vi "example.vi"() -> ()   [LabVIEW 2025, in "Dynamic-System.lvclass"]
uses:
  Dynamic-System.lvclass
  controller selection.ctl
panel:
  out "XY Graph":cluster{"Time":dbl[], "Reference":dbl[]}[](graph)
  in  "stop":bool
  out "error out":errorcluster
  out "Dynamic-System out":refnum<class "Dynamic-System.lvclass">
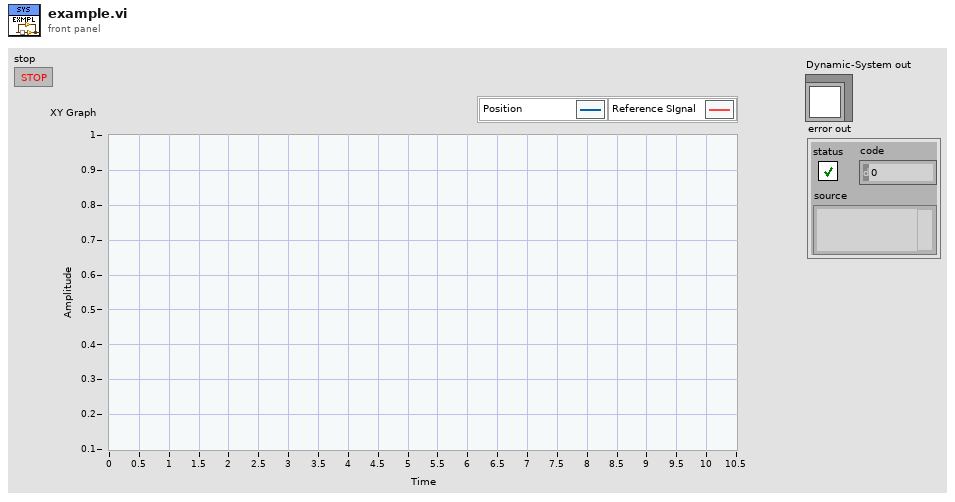
[diagram p1: front panel]
types:
  T1 = typedef "controller selection.ctl" = enum16{"No Control", "PID", "On Off"}
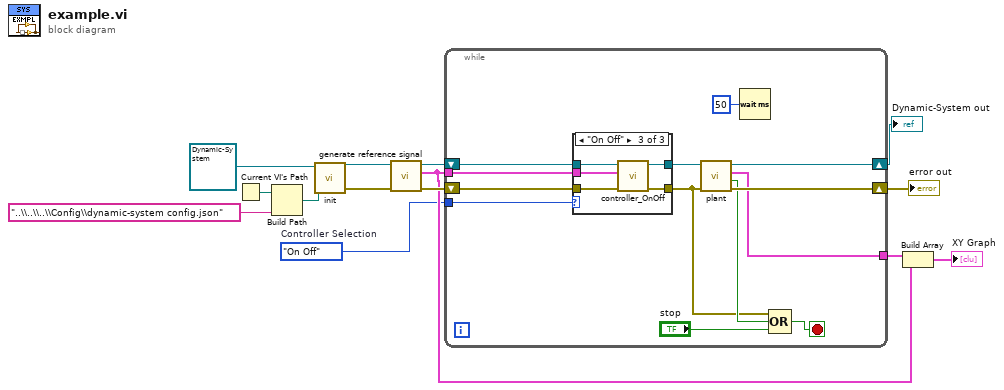
[diagram p0: block diagram]
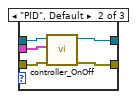
[diagram p3: hidden frame]
diagram:
  w1 = controller_selection."On Off"  # Controller Selection
  n1 = Current VI's Path() -> (path=w11:path)
  n2 = Build Path(base path=w11, name or relative path="..\\..\\..\\Config\\dynamic-system config.json") -> (appended path=w10:path)
  n3 = call-dynamic "init.vi"("Config Path"=w10, "Dynamic-System in"=refnum<class "Dynamic-System.lvclass"> refnum ("Dynamic-System.lvclass")) -> ("error out"=w7:errorcluster, "Dynamic-System out"=w8:refnum<class "Dynamic-System.lvclass">)  [unwired: 8 in]
  n4 = call-dynamic "generate reference signal.vi"("error in (no error)"=w7, "Dynamic-System in"=w8) -> ("error out"=w5:errorcluster, "Reference Array"=w2:cluster{"Time":dbl[], "Reference":dbl[]}, "Dynamic-System out"=w6:refnum<class "Dynamic-System.lvclass">)  [unwired: 7 in]
  n5 = while {
    shift-right: [w27] -> w14
    shift-left: w6 -> [w23]
    shift-right: [w26] -> w13
    shift-left: w5 -> [w22]
    tunnel: [w24] -> w4
    tunnel: w2 -> [w21]
    tunnel: w1 -> [w19]
    stop <- w15 stop-if-true
    n6 = case shown="\"On Off\"" w19 {
      tunnel: w23 -> [w29 w34 w39]
      tunnel: w22 -> [w28 w33 w38]
      tunnel: w21 -> [_ w30 w37]
      tunnel: [w29 w32 w36] -> w20
      tunnel: [w28 w31 w35] -> w16
      frame "No Control" {
      }
      frame "PID", Default {
        n7 = call-dynamic "controller_OnOff.vi"("error in (no error)"=w33, "Reference Array"=w30, "Dynamic-System in"=w34) -> ("error out"=w31:errorcluster, "Dynamic-System out"=w32:refnum<class "Dynamic-System.lvclass">)  [unwired: 7 in]
      }
      frame "On Off" {
        n8 = call-dynamic "controller_OnOff.vi"("error in (no error)"=w38, "Reference Array"=w37, "Dynamic-System in"=w39) -> ("error out"=w35:errorcluster, "Dynamic-System out"=w36:refnum<class "Dynamic-System.lvclass">)  [unwired: 7 in]
      }
    }
    n9 = call-dynamic "plant.vi"("error in (no error)"=w16, "Dynamic-System in"=w20) -> ("error out"=w26:errorcluster, "End of Simulation?"=w17:bool, "output cluster"=w24:cluster{"Time":dbl[], "State 1":dbl[]}, "Dynamic-System out"=w27:refnum<class "Dynamic-System.lvclass">)  [unwired: 6 in]
    n10 = Wait (ms)(milliseconds to wait=u32 50) -> ()  [unwired: 1 out]
    n11 = Compound Arithmetic op=OR(w16, w17, "stop") -> (w15:bool)
  }
  "Dynamic-System out" <- w14
  "error out" <- w13
  n12 = Build Array(w4, w2) -> (→"XY Graph":cluster{"Time":dbl[], "Reference":dbl[]}[])
